vi "Help setup.vi"() -> ()   [LabVIEW 2018]
panel:
  out "EN help":string="CONFIGURATION MANAGEMENT\n-By default, the configuration is loaded from the S4ICS.log file when starting the program. If S4ICS.log does not exist in the program folder, it will be created with default settings. To start the program using the configuration from another file (e.g. ECHARPE.log) use the command line \"S4ICS ECHARPE\".\n-\"CONFIG FILE\" shows the loaded file name and LAST CONFIGURATION the user and last modification date.\n-When saving with \"SAVE & LOGOUT\", the new configuration is inserted in this file. By clicking RETURN the configuration changes are discarded. -When saving with \"SAVE AS\", the program asks for a file name (existing or to be created) and the original setting is not changed.\n\nPERMISSIONS\n-Each user is given a permission between Start/Stop, Admin and Control. \n-With any permission you can start and stop the S4ICS TCP/IP server serving external clients (S4GUI) and through ASSIST test (CHECK) the mechanisms and put the mechanisms in the resting position (PARK). \n-The Control permission allows, exclusively, through CONTROL, to access advanced motor control functions.\n-Only the Admin permission allows you to change the configuration and manage S4ICS users. \n-As long as there is no user with Admin permission, S4ICS takes no action.\n\nUSER MANAGEMENT\nDelete: Select the user (<-, ->) and click Delete.\nInclusion: Type the name (and permission) and click Insert. The password will be requested and stored on the user's first login. PW indicates if the user already has a password.\nPassword change: Delete and re-add the user.\nPermission Change: Set Permission and click Change.\nAdmin permission is limited to 2 users only.\n\nEMAIL\n-If Email service is enabled, the Maintenance email will receive error notifications and the Configuration email will receive the data of the saved settings.\n-Regardless of the status of the Email service, CHECK SERVICE allows you to check if the email service is working,\n\nTIMEOUT\nAfter no user activity during \"Auto Logout period\", a new LOGIN will be necessary. If the timeout occurs while the program still has the default configuration, the program will be terminated." caption="INSTANT HELP"
  out "PT help":string="GERENCIAMENTO DE CONFIGURAÇÃO\n-Por default, a configuração é carregada do arquivo S4ICS.log ao iniciar o programa. Se S4ICS.log não exixtir na pasta do programa, ele será criado com as configurações default. Para iniciar o programa usando a configuração de outro arquivo (e.g. ECHARPE.log) use a linha de comando \"S4ICS ECHARPE\". \n-\"CONFIG FILE\" mostra o nome do arquivo carregado e LAST CONFIGURATION o usuário e a data da última modificação.\n-Ao salvar com \"SAVE & LOGOUT\", a nova configuração é inserida nesse arquivo. Ao clicar RETURN as modificações de configuração são descartadas. \n-Ao salvar com \"SAVE AS\", o programa solicita um nome de arquivo (existente ou a ser criado) e a configuração original não é alterada.  \n\nPERMISSÕES\n-Cada usuário recebe uma permissão entre Start/Stop, Admin e Control. \n-Com qualquer permissão se pode iniciar e parar o servidor TCP/IP do S4ICS que atende clientes externos (S4GUI) e por meio de ASSIST testar (CHECK) os mecanismos e colocar os mecanismos na posição de repouso (PARK). \n-A permissão Control permite, exclusivamente, por meio de CONTROL acessar funções avançadas de controle dos motores.\n-Somente a permissão Admin permite alterar a configuração e gerenciar usários do S4ICS. -Enquanto não houver um usuário com permissão Admin, o S4ICS não executa nenhuma ação.\n\nGERENCIAMENTO DE USUÁRIOS\n-Exclusão: \nSelecione o usuário (<-, ->) e clique Delete.\n-Inclusão: \nDigite o nome (e a permissão) e clique Insert. A senha será solicitada e armazenada no primeiro acesso do usuário. PW indica se o usuário já tem senha.\n-Troca de senha:\nExclua e inclua novamente o usuário.\n-Troca de permissão:\nAjuste Permission e clique Change. \nA permissão Admin está limitada a 2 usuários.\n\nE-MAIL\n-Se Email service estiver habilitado, o e-mail Maintenance receberá notificações de erro e o \ne-mail Configuration os dados das configurações que forem salvas.\n-Independete do estado de Email service, CHECK SERVICE permite verificar se o serviço de e-mail está funcionando,\n\nTIMEOUT\nApós o tempo \"Auto Logout period\" sem atividade do usuário, um novo LOGIN será necessário. Se o timeout ocorrer enquanto o programa ainda estiver com a configuração padrão, o programa será encerrado." caption="BREVE AJUDA"
  in  "ok":bool
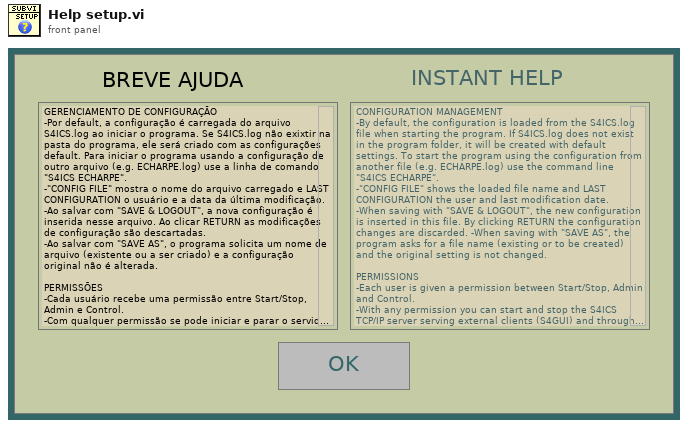
[diagram p1: front panel]
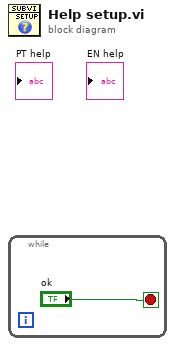
[diagram p0: block diagram]
diagram:
  n1 = while {
    stop <- "ok" stop-if-true
  }
